vi "test_VI Set-Get Protocol AKRSxxx.vi"(8 "error in (no error)":errorcluster, 11 "TestCase in":refnum<class "Instrument Addon Scripting API Custom Device Unit Tests.lvclass">) -> (0 "error out":errorcluster, 3 "TestCase out":refnum<class "Instrument Addon Scripting API Custom Device Unit Tests.lvclass">)   [LabVIEW 2018, in "Instrument Addon Scripting API Custom Device Unit Tests.lvclass"]
uses:
  Instrument Addon Scripting API Custom Device Unit Tests.lvclass
  Addon/Support Libraries/Protocols.lvlibp/AK RS-xxx/AK RS-xxx.lvclass
  C:/Users/nitest/Git/NI VS Instrument Addon Fork/Source/Addon/Support Libraries/Protocols.lvlibp/RS-xxx/RS-xxx.lvclass
  C:/Users/nitest/Git/NI VS Instrument Addon Fork/Source/Addon/Support Libraries/Protocols.lvlibp/Protocol Parent/Protocol Parent.lvclass
  NationalInstruments.VeriStand.SystemDefinitionAPI
  Addon/Support Libraries/Protocols.lvlibp/RS-xxx/Data Access/Write PortSettings.vi
  Instrument Addon Scripting API Test Assets/Instrument Addon Scripting API Test Assets.lvclass
  <vilib>/addons/_JKI Toolkits/VI Tester/TestCase.llb/TestCase.lvclass
  APIs/Scripting API/Instrument Addon Scripting API.lvlib
  C:/Program Files (x86)/National Instruments/LabVIEW 2018/vi.lib/addons/_JKI Toolkits/VI Tester/TestCase.llb/TestCase.lvclass
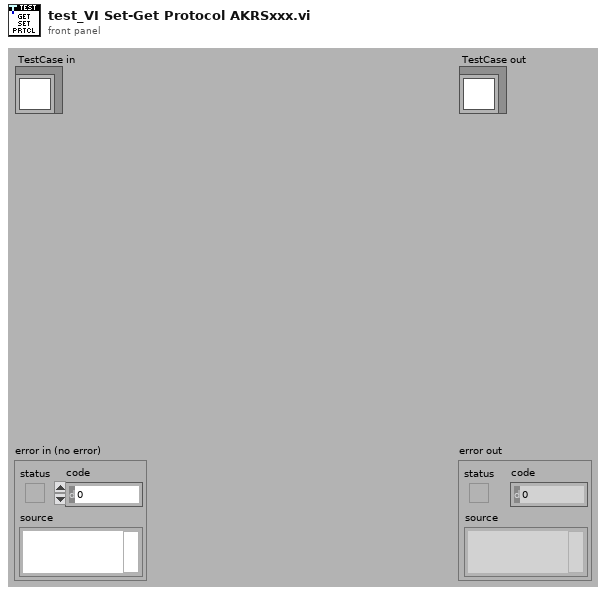
[diagram p1: front panel]
types:
  T1 = enum16{"NUL", "SOH", "STX", "ETX", "EOT", "ENQ", "ACK", "BEL", "BS", "HT", "LF", "VT", "FF", "CR", "SO", "SI", "DLE", "DC1", "DC2", "DC3", "DC4", "NAK", "SYN", "ETB", "CAN", "EM", "SUB", "ESC", "FS", "GS", "RS", "US", "SP", "!", "\"", "#", "$", "%", "&", "'", "(", ")", "*", "+", ",", "- (-)", ".", "/", "0", "1", "2", "3", "4", "5", "6", "7", "8", "9", ":", ";", "<", "=", ">", "?", "@", "A", "B", "C", "D", "E", "F", "G", "H", "I", "J", "K", "L", "M", "N", "O", "P", "Q", "R", "S", "T", "U", "V", "W", "X", "Y", "Z", "[", "\\", "]", "^", "_", "`", "a", "b", "c", "d", "e", "f", "g", "h", "i", "j", "k", "l", "m", "n", "o", "p", "q", "r", "s", "t", "u", "v", "w", "x", "y", "z", "{", "|", "}", "~"}
  T2 = cluster{"Port":string, "Baud Rate":u32, "Data Bits":u16, "Parity":enum16{"None", "Odd", "Even", "Mark", "Space"}, "Stop Bits":u16, "Flow Control":u16, "XON":enum16{"NUL", "SOH", "STX", "ETX", "EOT", "ENQ", "ACK", "BEL", "BS", "HT", "LF", "VT", "FF", "CR", "SO", "SI", "DLE", "DC1", "DC2", "DC3", "DC4", "NAK", "SYN", "ETB", "CAN", "EM", "SUB", "ESC", "FS", "GS", "RS", "US", "SP", "!", "\"", "#", "$", "%", "&", "'", "(", ")", "*", "+", ",", "- (-)", ".", "/", "0", "1", "2", "3", "4", "5", "6", "7", "8", "9", ":", ";", "<", "=", ">", "?", "@", "A", "B", "C", "D", "E", "F", "G", "H", "I", "J", "K", "L", "M", "N", "O", "P", "Q", "R", "S", "T", "U", "V", "W", "X", "Y", "Z", "[", "\\", "]", "^", "_", "`", "a", "b", "c", "d", "e", "f", "g", "h", "i", "j", "k", "l", "m", "n", "o", "p", "q", "r", "s", "t", "u", "v", "w", "x", "y", "z", "{", "|", "}", "~"}, "XOFF":enum16{"NUL", "SOH", "STX", "ETX", "EOT", "ENQ", "ACK", "BEL", "BS", "HT", "LF", "VT", "FF", "CR", "SO", "SI", "DLE", "DC1", "DC2", "DC3", "DC4", "NAK", "SYN", "ETB", "CAN", "EM", "SUB", "ESC", "FS", "GS", "RS", "US", "SP", "!", "\"", "#", "$", "%", "&", "'", "(", ")", "*", "+", ",", "- (-)", ".", "/", "0", "1", "2", "3", "4", "5", "6", "7", "8", "9", ":", ";", "<", "=", ">", "?", "@", "A", "B", "C", "D", "E", "F", "G", "H", "I", "J", "K", "L", "M", "N", "O", "P", "Q", "R", "S", "T", "U", "V", "W", "X", "Y", "Z", "[", "\\", "]", "^", "_", "`", "a", "b", "c", "d", "e", "f", "g", "h", "i", "j", "k", "l", "m", "n", "o", "p", "q", "r", "s", "t", "u", "v", "w", "x", "y", "z", "{", "|", "}", "~"}, "End Read on Termination Character":bool, "End Write on Termination Character":bool, "Termination Character":u8}
  T3 = typedef "Custom Device API.lvlib/Custom Device Item Ref.ctl" = u64
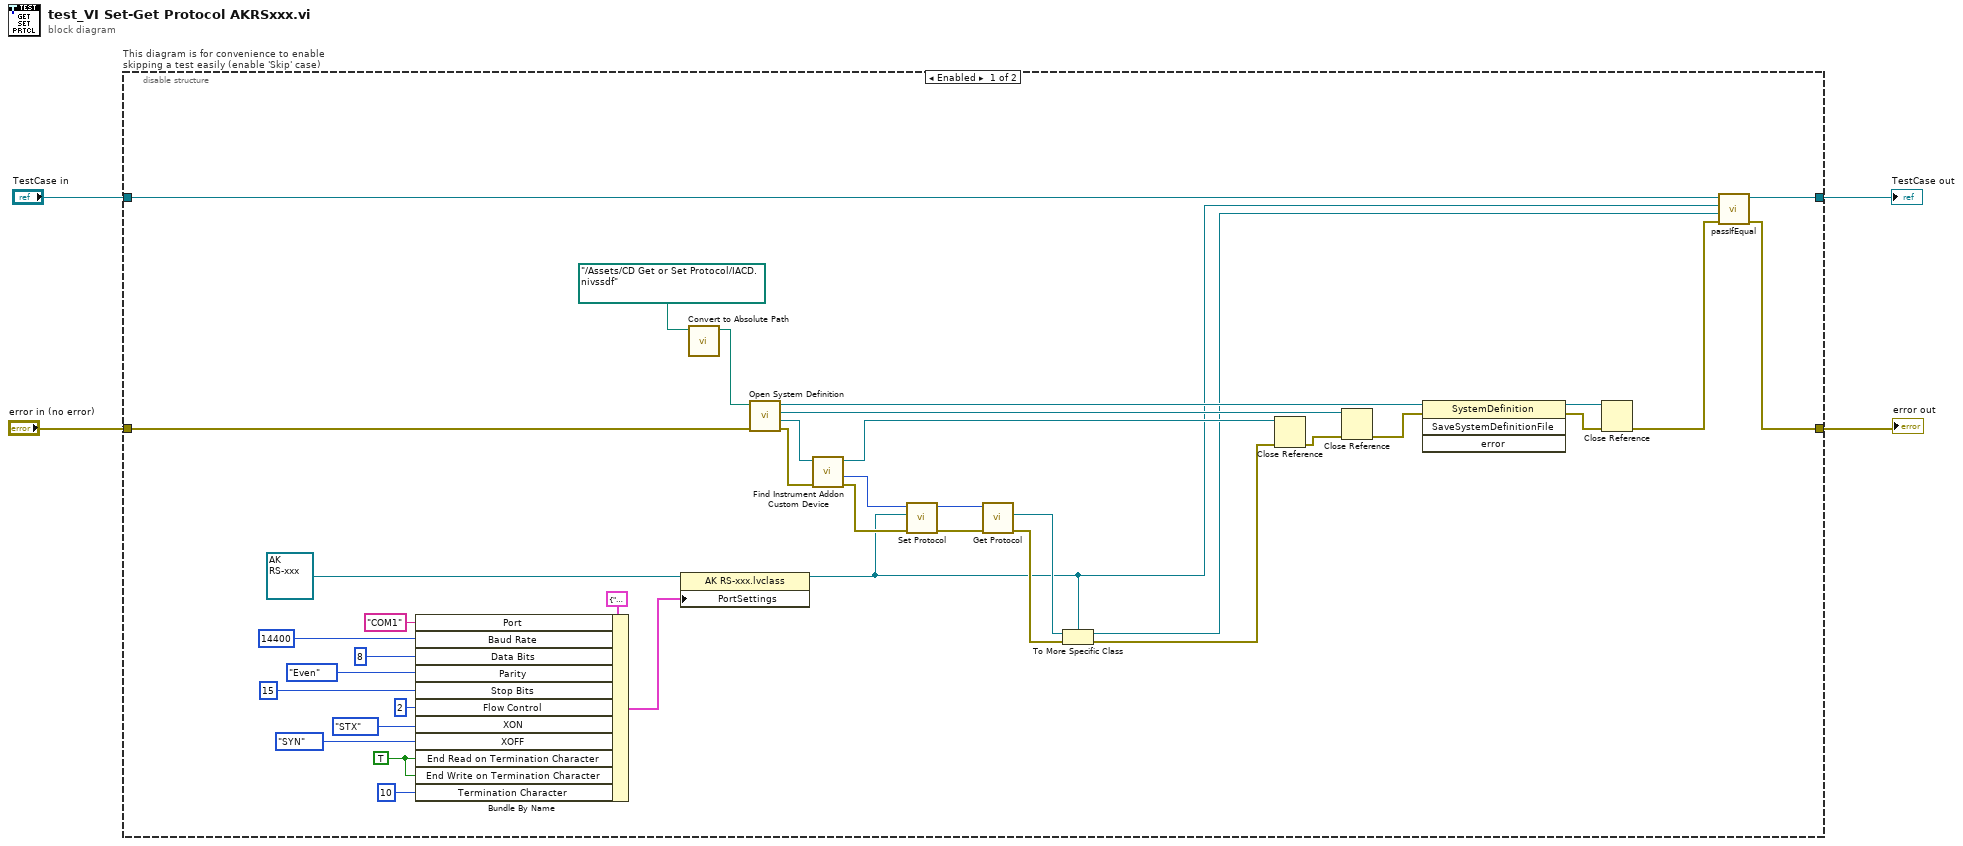
[diagram p0: block diagram]
diagram:
  n1 = disable-structure "This diagram is for convenience to enable skipping a test easily (enable 'Skip' case)" shown="Enabled" {
    disable-tunnel: "TestCase in" -> [w23 w46]
    disable-tunnel: [w22 w44] -> w1
    disable-tunnel: [w18 w45] -> w3
    disable-tunnel: "error in (no error)" -> [w42 w43]
    frame Enabled {
      w7 = TRUE ("End Read on Termination Character")
      n2 = Bundle By Name(cluster=T2 {"Port"="COM1", "Baud Rate"=9600, "Data Bits"=8, "Parity"=enum."None", "Stop Bits"=10, "Flow Control"=0, "XON"=enum."DC1", "XOFF"=enum."DC3", "End Read on Termination Character"=TRUE, "End Write on Termination Character"=TRUE, "Termination Character"=10} ("PortSettings"), "Port"="COM1", "Baud Rate"=u32 14400, "Data Bits"=u16 8, "Parity"=enum16{"None", "Odd", "Even", "Mark", "Space"}."Even", "Stop Bits"=u16 15, "Flow Control"=u16 2, "XON"=T1."STX", "XOFF"=T1."SYN", "End Read on Termination Character"=w7, "End Write on Termination Character"=w7, "Termination Character"=u8 10) -> (w16:T2)
      n3 = property class="AK RS-xxx.lvclass"(reference=refnum<class "AK RS-xxx.lvclass"> refnum ("Protocols.lvlibp:AK RS-xxx.lvclass"), "PortSettings"=w16) -> (reference out=w20:refnum<class "AK RS-xxx.lvclass">)  [unwired: 1 in, 1 out]
      n4 = call "Convert to Absolute Path.vi"("System Definition File"=path "../Assets/CD Get or Set Protocol/IACD.nivssdf" ("SDF file")) -> ("Absolute Path"=w40:path)  [unwired: 10 in]
      n5 = call "Open System Definition.vi"("error in (no error)"=w42, "System Definition File"=w40) -> ("error out"=w37:errorcluster, "Target Refnum"=w36:refnum<k24>, "Root Refnum"=w39:refnum<k24>, "System Definition Refnum"=w30:refnum<k24>)  [unwired: 6 in]
      n6 = call "Find Instrument Addon Custom Device.vi"("error in"=w37, "target in"=w36) -> ("error out"=w35:errorcluster, "NodeID"=w34:u64, "target out"=w33:refnum<k24>)  [unwired: 7 in]
      n7 = call "Set Protocol.vi"("Error In"=w35, "Protocol in"=w20, "Instrument Addon Refnum In"=w34) -> ("Error Out"=w31:errorcluster, "Instrument Addon Refnum Out"=w32:T3)  [unwired: 7 in]
      n8 = call "Get Protocol.vi"("Error In"=w31, "Instrument Addon Refnum In"=w32) -> ("Error Out"=w25:errorcluster, "Protocol"=w26:refnum<class "Protocol Parent.lvclass">)  [unwired: 7 in, 1 out]
      n9 = To More Specific Class(target class=w20, reference=w26, error in=w25) -> (specific class reference=w21:refnum<class "AK RS-xxx.lvclass">, error out=w24:errorcluster)
      n10 = Close Reference(reference=w33, error in (no error)=w24) -> (error out=w38:errorcluster)
      n11 = Close Reference(reference=w39, error in (no error)=w38) -> (error out=w29:errorcluster)
      n12 = invoke class="SystemDefinition" method="SaveSystemDefinitionFile"(reference=w30, error in=w29) -> (reference out=w28:refnum<k24>, error out=w27:errorcluster)  [unwired: 2 in, 2 out]
      n13 = Close Reference(reference=w28, error in (no error)=w27) -> (error out=w19:errorcluster)
      n14 = call-dynamic "passIfEqual.vi"("error in (no error)"=w19, "y"=w21, "x"=w20, "TestCase in"=w23) -> ("error out"=w18:errorcluster, "TestCase out"=w22:refnum<class "Instrument Addon Scripting API Custom Device Unit Tests.lvclass">)  [unwired: 6 in]
    }
    frame Disabled {
      # "skip test result while test is under development"
      n15 = call <vilib>:"skip.vi"("error in (no error)"=w43, "TestCase in"=w46) -> ("error out"=w45:errorcluster, "TestCase out"=w44:refnum<class "Instrument Addon Scripting API Custom Device Unit Tests.lvclass">)  [unwired: 8 in]
    }
  }
  "error out" <- w3
  "TestCase out" <- w1
